vi "Write Card refnum.vi"(8 "error in (no error)":errorcluster, 10 "Card refnum":refnum<vi>, 11 "Power Meter Display in":refnum<class "Power Meter Display.lvclass">) -> (0 "error out":errorcluster, 3 "Power Meter Display out":refnum<class "Power Meter Display.lvclass">)   [LabVIEW 2012, in "Display Panel.lvlib" / "Power Meter Display.lvclass"]
uses:
  Power Meter Display.lvclass
  Power Meter Display.lvclass/Power Meter Display.ctl
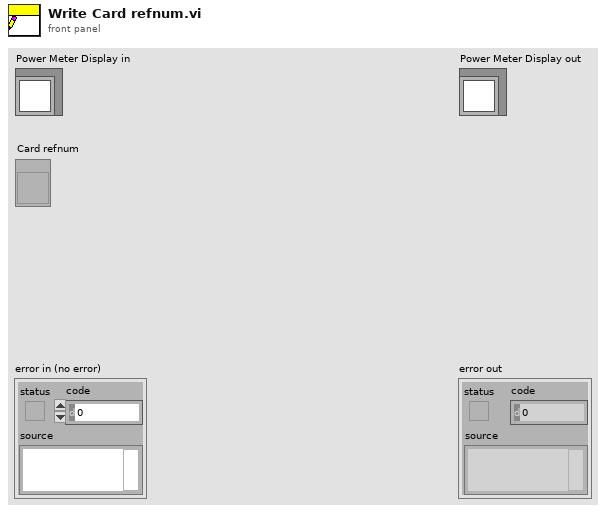
[diagram p1: front panel]
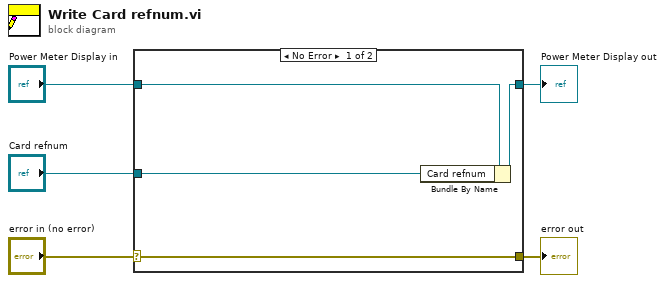
[diagram p0: block diagram]
diagram:
  n1 = case shown="No Error" "error in (no error)" {
    selector: "error in (no error)" -> [w9 w10]
    tunnel: [w9 w10] -> w4
    tunnel: [w7 w11] -> w2
    tunnel: "Power Meter Display in" -> [w8 w11]
    tunnel: "Card refnum" -> [w6 _]
    frame No Error {
      n2 = Bundle By Name(cluster=w8, "Card refnum"=w6) -> (w7:refnum<class "Power Meter Display.lvclass">)
    }
    frame Error {
    }
  }
  "error out" <- w4
  "Power Meter Display out" <- w2
